vi "Test1.vi"(8 "Numeric 2":dbl, 10 "Boolean":bool, 11 "Numeric":dbl) -> (1 "Meter":dbl(knob) scale=0.0..10.0)   [LabVIEW 2014]
panel:
  # "Adds the two numbers if Boolean is true, otherwise uses Pith. Rule."
  # "You could add something simple for testing"
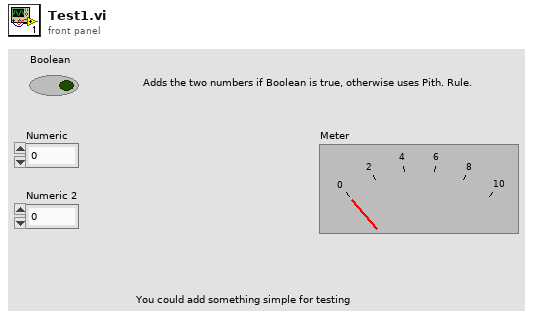
[diagram p1: front panel]
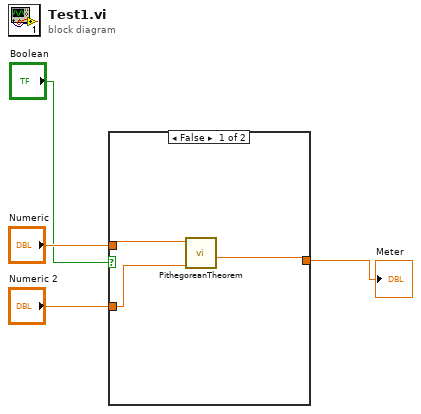
[diagram p0: block diagram]
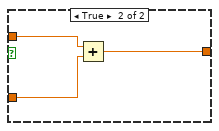
[diagram p2: hidden frame]
diagram:
  n1 = case shown="False" "Boolean" {
    tunnel: "Numeric" -> [w6 w10]
    tunnel: "Numeric 2" -> [w5 w9]
    tunnel: [w7 w8] -> w2
    frame False {
      n2 = call "PithegoreanTheorem.vi"("b"=w5, "a"=w6) -> ("c"=w7:dbl)  [unwired: 9 in]
    }
    frame True {
      n3 = Add(x=w10, y=w9) -> (x+y=w8:dbl)
    }
  }
  "Meter" <- w2
